vi "scale AI.vi"(7 "Voltage Range ch2":T1(ring), 10 "Ref-In":fxp<+/-,27,5>, 11 "gain":fxp<+,18,6>=1.0) -> (3 "signal":fxp<+/-,17,1>)   [LabVIEW 2018, in "tools.lvlib"]
uses:
  tools.lvlib
  <vilib>/rvi/FXPMathLib/FxpMul/XNode/nifxpmath_Multiplier.xnode
  <vilib>/rvi/FXPMathLib/sim/FxpSim.dll
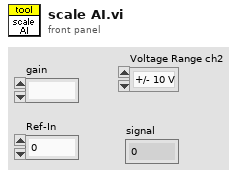
[diagram p1: front panel]
types:
  T1 = enum8{"+/- 10 V", "+/- 5 V", "+/- 2 V", "+/- 1 V"}
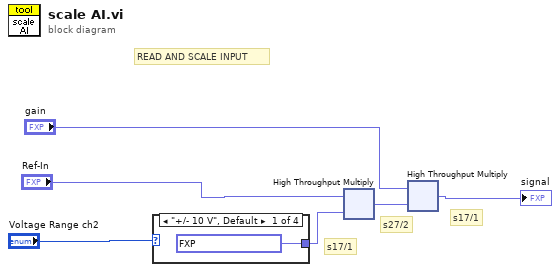
[diagram p0: block diagram]
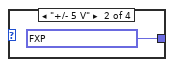
[diagram p2: hidden frame]
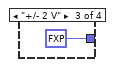
[diagram p3: hidden frame]
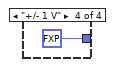
[diagram p4: hidden frame]
diagram:
  # "s17/1"
  # "s27/2"
  # "s17/1"
  # "READ AND SCALE INPUT"
  n1 = case shown="\"+/- 10 V\", Default" "Voltage Range ch2" {
    tunnel: [fxp<+,17,1> 0.100006103515625 ("y") fxp<+,17,1> 0.1999969482421875 ("y") fxp<+,17,1> 0.5 ("y") fxp<+,17,1> 1.0 ("y")] -> w6
    frame "+/- 10 V", Default {
    }
    frame "+/- 5 V" {
    }
    frame "+/- 2 V" {
    }
    frame "+/- 1 V" {
    }
  }
  n2 = xnode ("High Throughput Multiply")("x"="Ref-In", "y"=w6) -> ("x*y"=w5:fxp<+/-,27,2>)
  n3 = xnode ("High Throughput Multiply")("x"="gain", "y"=w5) -> ("x*y"=→"signal":fxp<+/-,17,1>)
